vi "New Assert Message.vi"(8 "error in (no error)":errorcluster, 10 "Assert Message":T1, 11 "Base Display Configuration in":refnum<class "Base Display Configuration.lvclass">) -> (0 "error out":errorcluster, 3 "Base Display Configuration out":refnum<class "Base Display Configuration.lvclass">)   [LabVIEW 2016, in "Assert API Components.lvlib" / "Assert Display.lvlib" / "Main Display.lvlib" / "Base Display Configuration.lvclass"]
uses:
  Base Display Configuration.lvclass
  Assert API Components/Message Data.ctl
  Assert API Components/Failure Actions.ctl
  Assert API Components/VI References.ctl
  Assert API Components/Assert API Components.lvlib
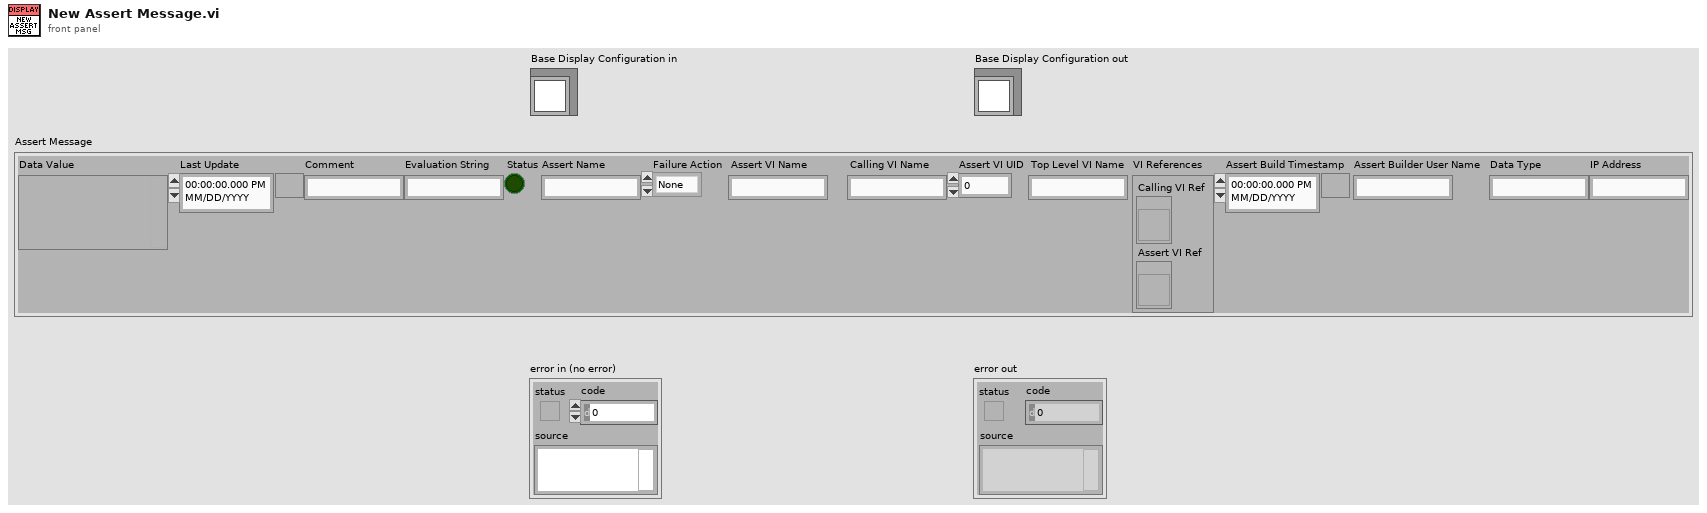
[diagram p1: front panel]
types:
  T1 = typedef "Assert API Components.lvlib/Message Data.ctl" = cluster{"Data Value":variant, "Last Update":timestamp, "Comment":string, "Evaluation String":string, "Status":bool, "Assert Name":string, "Failure Action":T2, "Assert VI Name":string, "Calling VI Name":string, "Assert VI UID":i32, "Top Level VI Name":string, "VI References":T3, "Assert Build Timestamp":timestamp, "Assert Builder User Name":string, "Data Type":string, "IP Address":string}
  T2 = typedef "Assert API Components.lvlib/Failure Actions.ctl" = enum16{"None", "Log To File", "Pause Execution", "Abort Execution"}
  T3 = typedef "Assert API Components.lvlib/VI References.ctl" = cluster{"Calling VI Ref":refnum<vi>, "Assert VI Ref":refnum<vi>}
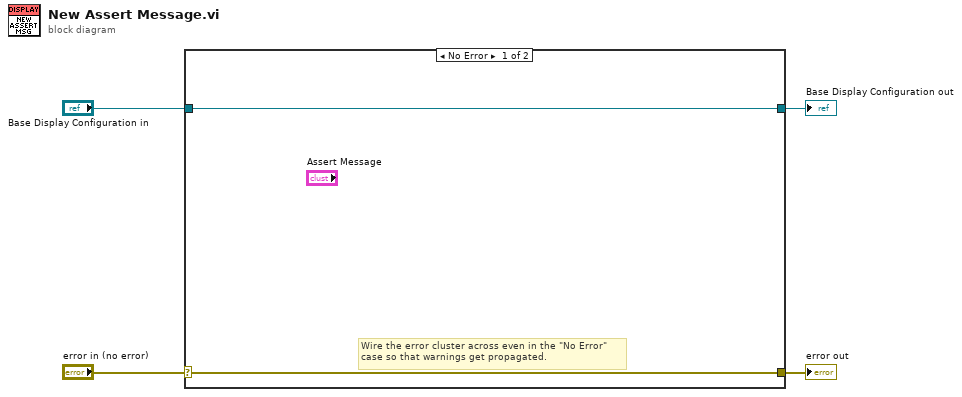
[diagram p0: block diagram]
diagram:
  n1 = case shown="No Error" "error in (no error)" {
    selector: "error in (no error)" -> [w5 w8]
    tunnel: [w5 w8] -> w3
    tunnel: [w6 w7] -> w1
    tunnel: "Base Display Configuration in" -> [w6 w7]
    frame No Error {
      # "Wire the error cluster across even in the \"No Error\"\ncase so that warnings get propagated."
    }
    frame Error {
    }
  }
  "error out" <- w3
  "Base Display Configuration out" <- w1
